vi "TtmDisconnect.vi"(3 "Ttm Name":string="TipTiltMirror[1]", 9 "error in (no error)":errorcluster) -> (6 "error out":errorcluster caption="error in (no error)")   [LabVIEW 2009]
uses:
  lib/lvrtc.dll
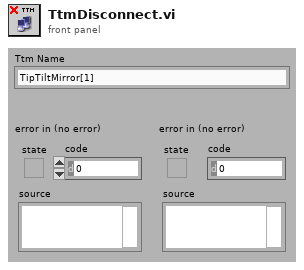
[diagram p1: front panel]
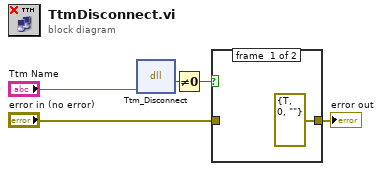
[diagram p0: block diagram]
diagram:
  n1 = dll-call lib="C:/Ohana/LV2009/OhanaOS-LV81/Instruments/RTC/Api/lib/lvrtc.dll" fn="Ttm_Disconnect"("TtmName"="Ttm Name") -> (w4:i32)  [unwired: 4 in, 2 out]
  n2 = Not Equal To 0?(x=w4) -> (x != 0?=w1:bool)
  n3 = case shown="False" w1 {
    tunnel: "error in (no error)" -> [_ w7]
    tunnel: [errorcluster {"status"=TRUE, "code"=0, "source"=""} ("error in (no error)") w7] -> w2
    frame #0 {
    }
    frame #1 {
    }
  }
  "error out" <- w2
